vi "Lidar Transform.vi"(10 "Transform Amount (mm)":dbl=-100.0 format="%#_13g", 11 "Pose":cluster{"X":dbl, "Y":dbl, "R":dbl}) -> (3 "Pose":cluster{"X":dbl, "Y":dbl, "R":dbl})   [LabVIEW 2018]
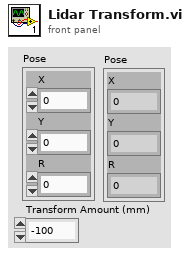
[diagram p1: front panel]
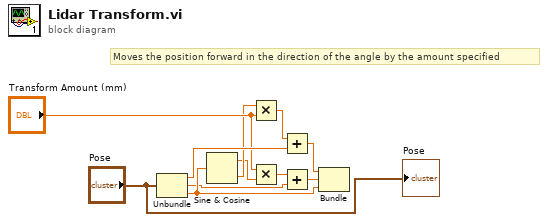
[diagram p0: block diagram]
diagram:
  # "Moves the position forward in the direction of the angle by the amount specified"
  n1 = Unbundle("Pose") -> ("X"=w6:dbl, "Y"=w7:dbl, "R"=w11:dbl)
  n2 = Sine & Cosine(0:w11) -> (1:w2:dbl, 2:w3:dbl)
  n3 = Multiply(x=w3, y="Transform Amount (mm)") -> (x*y=w5:dbl)
  n4 = Multiply(x="Transform Amount (mm)", y=w2) -> (x*y=w8:dbl)
  n5 = Add(x=w5, y=w6) -> (x+y=w9:dbl)
  n6 = Add(x=w8, y=w7) -> (x+y=w10:dbl)
  n7 = Bundle(w9, w10, "R"=w11) -> ()  [unwired: 1 in, 1 out]
  "Pose" <- "Pose"
